vi "PM-filter_waveform.vi"(10 "Addition signal to remove (0) [s]":dbl, 11 "waveform in":waveform(dbl)) -> (2 "data size (s)":dbl, 3 "waveform out":waveform(dbl))   [LabVIEW 2018]
uses:
  <vilib>/Analysis/3filter.llb/Filter Passband Type.ctl
  <vilib>/Analysis/3filter.llb/Butterworth Filter (DBL).vi
  <vilib>/Analysis/NI_AALBase.lvlib
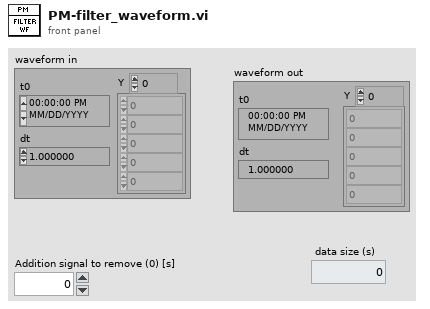
[diagram p1: front panel]
types:
  T1 = typedef "NI_AALBase.lvlib/Filter Passband Type.ctl" = enum32{"Lowpass", "Highpass", "Bandpass", "Bandstop"}
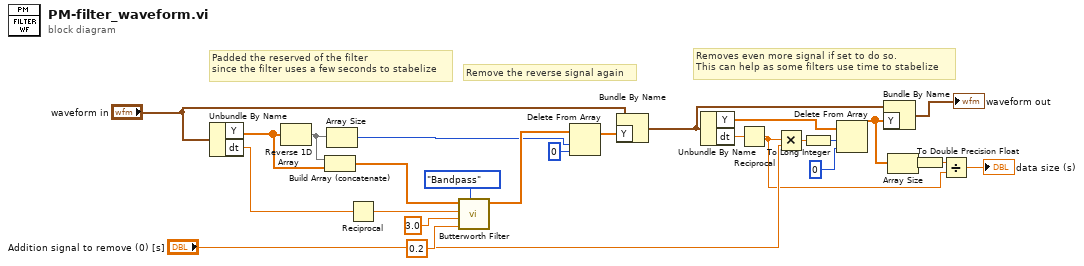
[diagram p0: block diagram]
diagram:
  # "Removes even more signal if set to do so.\nThis can help as some filters use time to stabelize"
  # "Remove the reverse signal again"
  # "Padded the reserved of the filter\nsince the filter uses a few seconds to stabelize"
  n1 = Unbundle By Name("waveform in") -> ("Y"=w22:dbl[], "dt"=w15:dbl)
  n2 = Reverse 1D Array(array=w22) -> (reversed array=w19:dbl[])
  n3 = Build Array (concatenate)(w19, w22) -> (w23:dbl[])
  n4 = Array Size(array=w19) -> (size(s)=w18:i32)
  n5 = Reciprocal(x=w15) -> (1/x=w14:dbl)
  n6 = call-poly <vilib>:"Butterworth Filter.vi"("filter type"=Filter_Passband_Type."Bandpass", "low cutoff freq: fl"=0.2, "high cutoff freq: fh"=3.0, "sampling freq: fs"=w14, "X"=w23) -> ("Filtered X"=w21:dbl[])  [unwired: 3 in, 1 out]
  n7 = Delete From Array(array=w21, length=w18, index=0) -> (array with subset deleted=w16:dbl[])  [unwired: 1 out]
  n8 = Bundle By Name(cluster="waveform in", "Y"=w16) -> (w11:waveform(dbl))
  n9 = Unbundle By Name(w11) -> ("Y"=w10:dbl[], "dt"=w9:dbl)
  n10 = Reciprocal(x=w9) -> (1/x=w1:dbl)
  n11 = Multiply(x=w1, y="Addition signal to remove (0) [s]") -> (x*y=w3:dbl)
  n12 = To Long Integer(number=w3) -> (32bit integer=w7:i32)
  n13 = Delete From Array(array=w10, length=w7, index=0) -> (array with subset deleted=w6:dbl[])  [unwired: 1 out]
  n14 = Bundle By Name(cluster=w11, "Y"=w6) -> (→"waveform out":waveform(dbl))
  n15 = Array Size(array=w6) -> (size(s)=w5:i32)
  n16 = To Double Precision Float(number=w5) -> (double precision float=w4:dbl)
  n17 = Divide(x=w4, y=w1) -> (x/y=→"data size (s)":dbl)
